vi "Supercell Structure into a Box.vi"(7 "Max # of atoms":i32=9999999, 8 "Keep old lattice vectors?":bool, 9 "Center Subcrystal":bool, 10 "Draw Box":T2, 11 "Subcrystal":T1={"Structure Name"="Gamm8 Subcrystal", "Lattice vector a"=[2.3379684769090283, 4.050155798593294, -3.073453095936429e-05], "Lattice vector b"=[0.0, 2.7000749366574968, 3.8175198422845327], "Lattice vector c"=[4.675927601962877, 0.0, 0.0], "Atoms Array"=[{"Atom Name"="Cd", "Positions (Direct)"=[[0.0, 2.2797955771e-06, 0.2499966378910753]], "Positions (Cartesian)"=[[0.0, -3.2294507389786483e-06, 2.863111017657439]]}, {"Atom Name"="Te", "Positions (Direct)"=[[0.0, -2.2797955771e-06, 3.3621089247e-06]], "Positions (Cartesian)"=[[0.0, -1.5237858666867705e-05, -2.8630725126350507]]}], "# of atoms"=2} {"Atoms Array"."Positions (Cartesian)" format="%#_4f"; "Atoms Array"."Positions (Direct)" format="%#_4f"}) -> (0 "error out":errorcluster, 2 "Supercells Filled":dbl[][](array[numeric]), 3 "Expanded cubic Structure":T1={"Structure Name"="Gamm8 Subcrystal", "Lattice vector a"=[2.3379684769090283, 4.050155798593294, -3.073453095936429e-05], "Lattice vector b"=[0.0, 2.7000749366574968, 3.8175198422845327], "Lattice vector c"=[4.675927601962877, 0.0, 0.0], "Atoms Array"=[{"Atom Name"="Cd", "Positions (Direct)"=[[0.0, 2.2797955771e-06, 0.2499966378910753]], "Positions (Cartesian)"=[[0.0, -3.2294507389786483e-06, 2.863111017657439]]}, {"Atom Name"="Te", "Positions (Direct)"=[[0.0, -2.2797955771e-06, 3.3621089247e-06]], "Positions (Cartesian)"=[[0.0, -1.5237858666867705e-05, -2.8630725126350507]]}], "# of atoms"=2} {"Atoms Array"."Positions (Cartesian)" format="%#_4f"; "Atoms Array"."Positions (Direct)" format="%#_4f"})   [LabVIEW 2010]
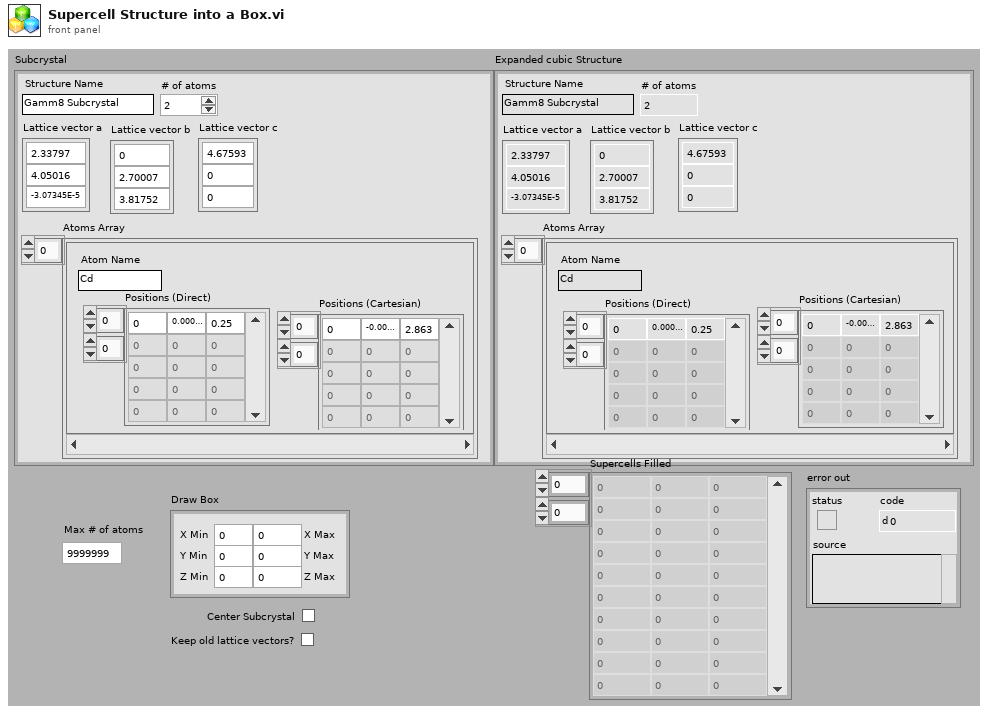
[diagram p1: front panel]
types:
  T1 = cluster{"Structure Name":string, "Lattice vector a":dbl[], "Lattice vector b":dbl[], "Lattice vector c":dbl[], "Atoms Array":cluster{"Atom Name":string, "Positions (Direct)":dbl[][], "Positions (Cartesian)":dbl[][]}[], "# of atoms":i32}
  T2 = cluster{"X Min":dbl, "X Max":dbl, "Y Min":dbl, "Y Max":dbl, "Z Min":dbl, "Z Max":dbl}
  T3 = cluster{"Atom Name":string, "Positions (Direct)":dbl[][], "Positions (Cartesian)":dbl[][]}[]
  T4 = cluster{"Atom Name":string, "Positions (Direct)":dbl[][], "Positions (Cartesian)":dbl[][]}
  T5 = cluster{"Atom Name":string, "Positions (Direct)":dbl[][], "Output Array":dbl[][]}
  T6 = cluster{string, "Lattice vector a":dbl[], "Lattice vector b":dbl[], "Lattice vector c":dbl[], cluster{"Atom Name":string, "Positions (Direct)":dbl[][], "Output Array":dbl[][]}[], i32}
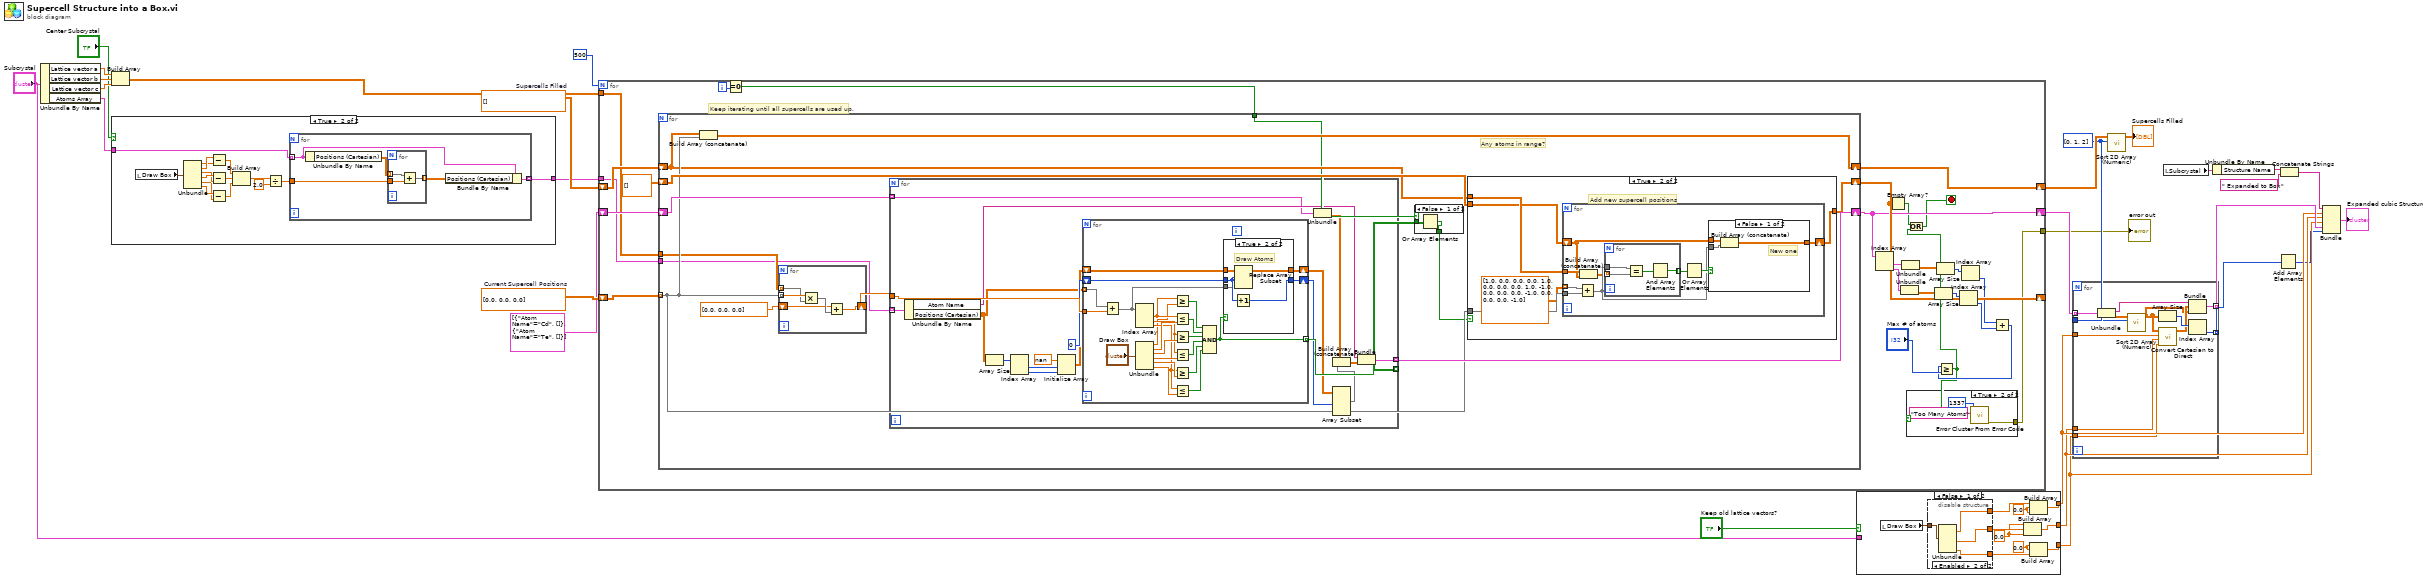
[diagram p0: block diagram]
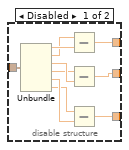
[diagram p2: hidden frame]
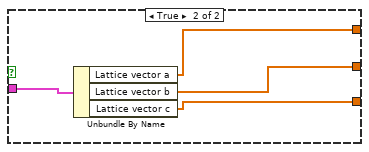
[diagram p3: hidden frame]
diagram:
  w15 = i32[] [0, 1, 2] ("Sort by Cols")
  w27 = dbl[][] []  # Supercells Filled
  w29 = dbl[][] [[0.0, 0.0, 0.0]]  # Current Supercell Positions
  n1 = Unbundle By Name("Subcrystal") -> ("Lattice vector a"=w25:dbl[], "Lattice vector b"=w24:dbl[], "Lattice vector c"=w23:dbl[], "Atoms Array"=w26:T3)
  n2 = Build Array(w25, w24, w23) -> (w22:dbl[][])
  n3 = case shown="True" "Center Subcrystal" {
    tunnel: w26 -> [w30 w45]
    tunnel: [w30 w31] -> w21
    frame False {
    }
    frame True {
      n4 = local read "Draw Box"() -> (w44:T2)
      n5 = Unbundle(w44) -> ("X Min"=w42:dbl, "X Max"=w43:dbl, "Y Min"=w39:dbl, "Y Max"=w40:dbl, "Z Min"=w36:dbl, "Z Max"=w37:dbl)
      n6 = Subtract(x=w43, y=w42) -> (x-y=w41:dbl)
      n7 = Subtract(x=w40, y=w39) -> (x-y=w38:dbl)
      n8 = Subtract(x=w37, y=w36) -> (x-y=w35:dbl)
      n9 = Build Array(w41, w38, w35) -> (w34:dbl[])
      n10 = Divide(x=w34, y=2.0) -> (x/y=w32:dbl[])
      n11 = for {
        tunnel: w45 -> [w48] mode=indexing
        tunnel: w32 -> [w49]
        tunnel: [w46] -> w31 mode=indexing
        n12 = Unbundle By Name(w48) -> ("Positions (Cartesian)"=w50:dbl[][])
        n13 = for {
          tunnel: w50 -> [w53] mode=indexing
          tunnel: w49 -> [w52]
          tunnel: [w51] -> w47 mode=indexing
          n14 = Add(x=w53, y=w52) -> (x+y=w51:dbl[])
        }
        n15 = Bundle By Name(cluster=w48, "Positions (Cartesian)"=w47) -> (w46:T4)
      }
    }
  }
  n16 = for {
    N: 500 -> [_]
    shift-right: [w71] -> _
    shift-left: w29 -> [w78]
    shift-right: [w68] -> w16
    shift-left: cluster{"Atom Name":string, dbl[][]}[] [{"Atom Name"="Cd", []}, {"Atom Name"="Te", []}] -> [w76]
    shift-right: [w74] -> w19
    shift-left: w27 -> [w75]
    tunnel: w22 -> [w73]
    tunnel: w21 -> [w72]
    tunnel: [w54] -> w1
    i -> [w70]
    stop <- w63 stop-if-true
    # "Keep iterating until all supercells are used up."
    n17 = Equal To 0?(x=w70) -> (x = 0?=w69:bool)
    n18 = for {
      shift-right: [w90] -> w71
      shift-left: dbl[][] [] ("Supercell Positions") -> [w93]
      tunnel: w78 -> [w89] mode=indexing
      shift-right: [w92] -> w68
      shift-left: w76 -> [w91]
      shift-right: [w85] -> w74
      shift-left: w75 -> [w88]
      tunnel: w73 -> [w87]
      tunnel: w72 -> [w86]
      tunnel: w69 -> [w82]
      # "Any atoms in range?"
      n19 = Build Array (concatenate)(w88, w89) -> (w85:dbl[][])
      n20 = for {
        tunnel: w89 -> [w126] mode=indexing
        shift-right: [w124] -> w94
        shift-left: dbl[] [0.0, 0.0, 0.0] -> [w123]
        tunnel: w87 -> [w122] mode=indexing
        n21 = Multiply(x=w126, y=w122) -> (x*y=w125:dbl[])
        n22 = Add(x=w123, y=w125) -> (x+y=w124:dbl[])
      }
      n23 = for {
        tunnel: w86 -> [w143] mode=indexing
        tunnel: w94 -> [w144]
        tunnel: [w142] -> w84 mode=indexing
        tunnel: w91 -> [w139] mode=indexing
        tunnel: [w140] -> w92 mode=indexing
        n24 = Unbundle By Name(w143) -> ("Atom Name"=w141:string, "Positions (Cartesian)"=w133:dbl[][])
        n25 = Array Size(array=w133) -> (size(s)=w132:i32[])
        n26 = Index Array(array=w132) -> (element #1=w131:i32, element #2=w130:i32)  [unwired: 2 in]
        n27 = Initialize Array(nan ("element"), w131, w130) -> (w134:dbl[][])
        n28 = for {
          tunnel: w133 -> [w168] mode=indexing
          tunnel: w144 -> [w167]
          shift-right: [w164] -> w129
          shift-left: w134 -> [w163]
          tunnel: [w162] -> w142 mode=indexing
          shift-right: [w160] -> w128
          shift-left: 0 -> [w161]
          n29 = Add(x=w168, y=w167) -> (x+y=w165:dbl[])
          n30 = Index Array(array=w165) -> (element #1=w159:dbl, element #2=w153:dbl, element #3=w147:dbl)  [unwired: 3 in]
          n31 = Unbundle("Draw Box") -> ("X Min"=w145:dbl, "X Max"=w158:dbl, "Y Min"=w155:dbl, "Y Max"=w152:dbl, "Z Min"=w150:dbl, "Z Max"=w148:dbl)
          n32 = Greater Or Equal?(x=w159, y=w145) -> (x >= y?=w157:bool)
          n33 = Less Or Equal?(x=w159, y=w158) -> (x <= y?=w156:bool)
          n34 = Greater Or Equal?(x=w153, y=w155) -> (x >= y?=w154:bool)
          n35 = Less Or Equal?(x=w153, y=w152) -> (x <= y?=w151:bool)
          n36 = Greater Or Equal?(x=w147, y=w150) -> (x >= y?=w149:bool)
          n37 = Less Or Equal?(x=w147, y=w148) -> (x <= y?=w146:bool)
          n38 = Compound Arithmetic op=AND(w157, w156, w154, w151, w149, w146) -> (w162:bool)
          n39 = case shown="True" w162 {
            tunnel: w165 -> [_ w172]
            tunnel: [w170 w171] -> w164
            tunnel: w163 -> [w170 w174]
            tunnel: w161 -> [w169 w173]
            tunnel: [w169 w175] -> w160
            frame False {
              # "Not inside box"
            }
            frame True {
              # "Draw Atoms"
              n40 = Increment(x=w173) -> (x+1=w175:i32)
              n41 = Replace Array Subset(array=w174, new element=w172, index (row)=w173) -> (w171:dbl[][])  [unwired: 1 in]
            }
          }
        }
        n42 = Unbundle(w139) -> (w137:dbl[][])  [unwired: 1 out]
        n43 = Array Subset(array=w129, length (row)=w128) -> (w127:dbl[][])  [unwired: 3 in]
        n44 = Build Array (concatenate)(w137, w127) -> (w136:dbl[][])
        n45 = Bundle("Atom Name"=w141, w136) -> (w140:cluster{"Atom Name":string, dbl[][]})  [unwired: 1 in]
      }
      n46 = case shown="False" w82 {
        selector: w82 -> [_ w98]
        tunnel: w84 -> [w97 _]
        tunnel: [w96 w98] -> w83
        frame False {
          n47 = Or Array Elements(Boolean array=w97) -> (logical OR=w96:bool)
        }
        frame True {
        }
      }
      n48 = case shown="True" w83 {
        tunnel: w89 -> [_ w104]
        tunnel: [w99 w100] -> w90
        tunnel: w93 -> [w99 w101]
        tunnel: w88 -> [_ w102]
        frame False {
          # "Don't sweat it"
        }
        frame True {
          # "Add new supercell positions"
          n49 = for {
            tunnel: w104 -> [w112]
            tunnel: dbl[][] [[1.0, 0.0, 0.0], [0.0, 1.0, 0.0], [0.0, 0.0, 1.0], [-1.0, 0.0, 0.0], [0.0, -1.0, 0.0], [0.0, 0.0, -1.0]] -> [w113] mode=indexing
            tunnel: w102 -> [w107]
            shift-right: [w111] -> w100
            shift-left: w101 -> [w106]
            n50 = Add(x=w113, y=w112) -> (x+y=w109:dbl[])
            n51 = Build Array (concatenate)(w107, w106) -> (w105:dbl[][])
            n52 = for {
              tunnel: w109 -> [w121]
              tunnel: w105 -> [w120] mode=indexing
              tunnel: [w118] -> w108 mode=indexing
              n53 = Equal?(x=w121, y=w120) -> (x = y?=w119:bool[])
              n54 = And Array Elements(Boolean array=w119) -> (logical AND=w118:bool)
            }
            n55 = Or Array Elements(Boolean array=w108) -> (logical OR=w110:bool)
            n56 = case shown="False" w110 {
              tunnel: w109 -> [w116 _]
              tunnel: [w115 w117] -> w111
              tunnel: w106 -> [w114 w117]
              frame False {
                # "New one"
                n57 = Build Array (concatenate)(w114, w116) -> (w115:dbl[][])
              }
              frame True {
                # "Already Did this one"
              }
            }
          }
        }
      }
    }
    n58 = Index Array(array=w68) -> (element #1=w67:cluster{"Atom Name":string, dbl[][]}, element #2=w59:cluster{"Atom Name":string, dbl[][]})  [unwired: 2 in]
    n59 = Empty Array?(array=w71) -> (empty?=w64:bool)
    n60 = Unbundle(w59) -> (w60:dbl[][])  [unwired: 1 out]
    n61 = Unbundle(w67) -> (w66:dbl[][])  [unwired: 1 out]
    n62 = Array Size(array=w60) -> (size(s)=w61:i32[])
    n63 = Array Size(array=w66) -> (size(s)=w65:i32[])
    n64 = Index Array(array=w61) -> (element=w57:i32)  [unwired: 1 in]
    n65 = Index Array(array=w65) -> (element=w58:i32)  [unwired: 1 in]
    n66 = Add(x=w58, y=w57) -> (x+y=w56:i32)
    n67 = Greater Or Equal?(x=w56, y="Max # of atoms") -> (x >= y?=w55:bool)
    n68 = case shown="True" w55 {
      tunnel: [_ w81] -> w54
      frame False {
      }
      frame True {
        n69 = call <vilib>:"Error Cluster From Error Code.vi"("error message (\"\")"="Too Many Atoms" ("error message (\"\")"), "error code (0)"=1337) -> ("error out"=w81:errorcluster)  [unwired: 7 in]
      }
    }
    n70 = Or(x=w64, y=w55) -> (x .or. y?=w63:bool)
  }
  "error out" <- w1
  n71 = case shown="False" "Keep old lattice vectors?" {
    tunnel: [w184 w202] -> w13
    tunnel: [w183 w201] -> w12
    tunnel: [w182 w200] -> w11
    tunnel: "Subcrystal" -> [_ w203]
    frame False {
      w177 = 0.0 ("element")
      w178 = 0.0 ("element")
      w181 = 0.0 ("element")
      n72 = local read "Draw Box"() -> (w185:T2)
      n73 = disable-structure shown="Enabled" {
        disable-tunnel: w185 -> [w195 w199]
        disable-tunnel: [w188 w198] -> w180
        disable-tunnel: [w187 w197] -> w179
        disable-tunnel: [w186 w196] -> w176
        frame Disabled {
          n74 = Unbundle(w195) -> ("X Min"=w190:dbl, "X Max"=w189:dbl, "Y Min"=w192:dbl, "Y Max"=w191:dbl, "Z Min"=w194:dbl, "Z Max"=w193:dbl)
          n75 = Subtract(x=w189, y=w190) -> (x-y=w188:dbl)
          n76 = Subtract(x=w191, y=w192) -> (x-y=w187:dbl)
          n77 = Subtract(x=w193, y=w194) -> (x-y=w186:dbl)
        }
        frame Enabled {
          n78 = Unbundle(w199) -> ("X Max"=w198:dbl, "Y Max"=w197:dbl, "Z Max"=w196:dbl)  [unwired: 3 out]
        }
      }
      n79 = Build Array(w178, w179, w178) -> (w183:dbl[])
      n80 = Build Array(w180, w181, w181) -> (w184:dbl[])
      n81 = Build Array(w177, w177, w176) -> (w182:dbl[])
    }
    frame True {
      n82 = Unbundle By Name(w203) -> ("Lattice vector a"=w202:dbl[], "Lattice vector b"=w201:dbl[], "Lattice vector c"=w200:dbl[])
    }
  }
  n83 = for {
    tunnel: w16 -> [w215] mode=indexing
    tunnel: w15 -> [w213]
    tunnel: [w211] -> w14 mode=indexing
    tunnel: w13 -> [w210]
    tunnel: w12 -> [w209]
    tunnel: w11 -> [w208]
    tunnel: [w206] -> w6 mode=indexing
    n84 = Unbundle(w215) -> ("Atom Name"=w212:string, w214:dbl[][])
    n85 = call "Sort 2D Array (Numeric).vi"("Sort by Cols"=w213, "Input Array"=w214) -> ("Output Array"=w204:dbl[][])  [unwired: 9 in]
    n86 = Array Size(array=w204) -> (size(s)=w207:i32[])
    n87 = call "Convert Cartesian to Direct.vi"("Lattice vector c"=w208, "Lattice vector b"=w209, "Lattice vector a"=w210, "Positions (Cartesian)"=w204) -> ("Positions (Direct)"=w205:dbl[][])  [unwired: 7 in]
    n88 = Bundle("Atom Name"=w212, "Positions (Direct)"=w205, "Output Array"=w204) -> (w211:T5)  [unwired: 1 in]
    n89 = Index Array(array=w207) -> (element=w206:i32)  [unwired: 1 in]
  }
  n90 = call "Sort 2D Array (Numeric).vi"("Sort by Cols"=w15, "Input Array"=w19) -> ("Output Array"=→"Supercells Filled":dbl[][])  [unwired: 9 in]
  n91 = local read "Subcrystal"() -> (w10:T1)
  n92 = Unbundle By Name(w10) -> ("Structure Name"=w9:string)
  n93 = Add Array Elements(numeric array=w6) -> (sum=w5:i32)
  n94 = Concatenate Strings(w9, " Expanded to Box" ("string")) -> (w7:string)
  n95 = Bundle(w7, "Lattice vector a"=w13, "Lattice vector b"=w12, "Lattice vector c"=w11, w14, w5) -> (→"Expanded cubic Structure":T6)  [unwired: 1 in]
